vi "Init Series Graph.vi"(6 "Z Scale.Marker Values[]":cluster{"Numeric":dbl, "Numeric":u32}[](array[cluster]), 7 "Graphs":T1, 8 "error in (no error)":errorcluster, 9 "Shots":u32, 10 "Image Size":cluster{"Height":u32, "Width":u32}, 11 "Series Graph in":refnum<class "Series Graph.lvclass">) -> (0 "error out":errorcluster, 3 "Series Graph out":refnum<class "Series Graph.lvclass">)   [LabVIEW 2023, in "Series Graph.lvclass"]
uses:
  Series Graph.lvclass
  Series Graph.lvclass/Series Graph.ctl
  Detail Graph/Detail Graph.lvclass
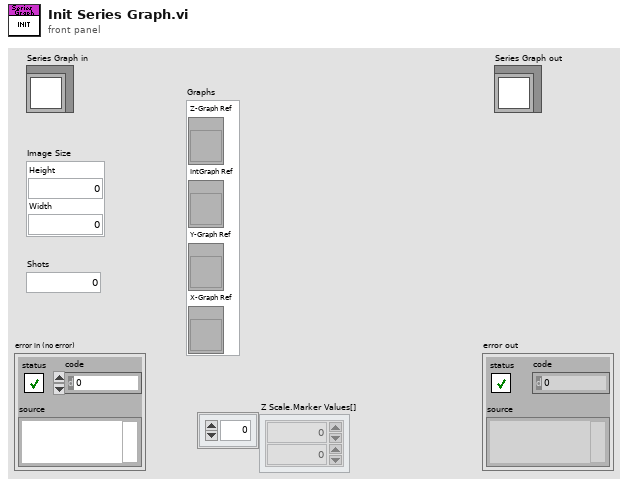
[diagram p1: front panel]
types:
  T1 = cluster{"Z-Graph Ref":refnum<vi>, "IntGraph Ref":refnum<vi>, "Y-Graph Ref":refnum<vi>, "X-Graph Ref":refnum<vi>}
  T2 = cluster{"IntGraph Ref":refnum<vi>, "Y-Graph Ref":refnum<vi>, "X-Graph Ref":refnum<vi>}
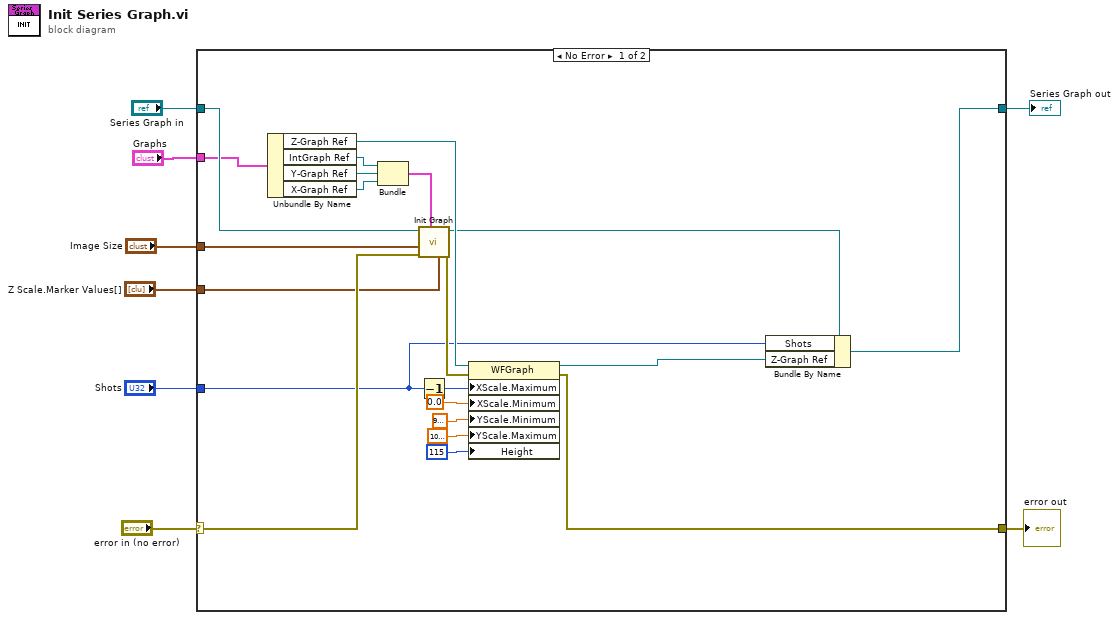
[diagram p0: block diagram]
diagram:
  n1 = case shown="No Error" "error in (no error)" {
    selector: "error in (no error)" -> [w29 w31]
    tunnel: [w9 w31] -> w7
    tunnel: [w10 w30] -> w2
    tunnel: "Series Graph in" -> [w28 w30]
    tunnel: "Image Size" -> [w21 _]
    tunnel: "Shots" -> [w12 _]
    tunnel: "Z Scale.Marker Values[]" -> [w27 _]
    tunnel: "Graphs" -> [w19 _]
    frame No Error {
      n2 = Unbundle By Name(w19) -> ("Z-Graph Ref"=w14:refnum<vi>, "IntGraph Ref"=w18:refnum<vi>, "Y-Graph Ref"=w17:refnum<vi>, "X-Graph Ref"=w16:refnum<vi>)
      n3 = Bundle("IntGraph Ref"=w18, "Y-Graph Ref"=w17, "X-Graph Ref"=w16) -> (w15:T2)  [unwired: 1 in]
      n4 = call "Init Graph.vi"("Z Scale.Marker Values[]"=w27, "Graphs"=w15, "error in (no error)"=w29, "Images Size"=w21, "Detail Graph.lvclass"=w28) -> ("error out"=w26:errorcluster, "Detail Graph out.lvclass"=w13:refnum<class "Series Graph.lvclass">)  [unwired: 5 in]
      n5 = Decrement(x=w12) -> (x-1=w20:u32)
      n6 = property class="WFGraph"(reference=w14, error in=w26, "XScale.Maximum"=w20, "XScale.Minimum"=0.0 ("X Scale.Range:Minimum"), "YScale.Minimum"=9000.0 ("Y Scale.Range:Minimum"), "YScale.Maximum"=10000.0 ("Y Scale.Range:Maximum"), "Height"=u32 115 ("Plot Area:Size:Height")) -> (reference out=w11:refnum<vi>, error out=w9:errorcluster)
      n7 = Bundle By Name(cluster=w13, "Shots"=w12, "Z-Graph Ref"=w11) -> (w10:refnum<class "Series Graph.lvclass">)
    }
    frame Error {
    }
  }
  "error out" <- w7
  "Series Graph out" <- w2
